vi "File.Sort Path Length, Long to Short.vi"(11 "Path Array":path[](array[path])) -> (3 "Path Array Out":path[](array[path]))   [LabVIEW 2018]
panel:
  # "Longest to Shortest"
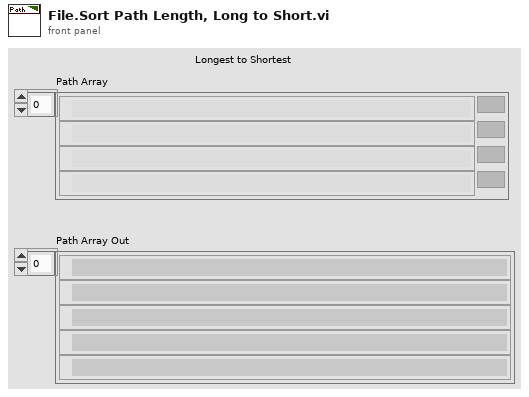
[diagram p1: front panel]
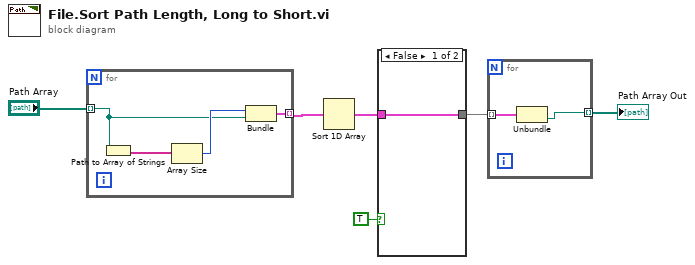
[diagram p0: block diagram]
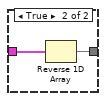
[diagram p2: hidden frame]
diagram:
  n1 = for {
    tunnel: "Path Array" -> [w8] mode=indexing
    tunnel: [w7] -> w5 mode=indexing
    n2 = Path to Array of Strings(0:w8) -> (2:w10:string[])  [unwired: 1 out]
    n3 = Array Size(array=w10) -> (size(s)=w9:i32)
    n4 = Bundle(w9, "Path"=w8) -> (w7:cluster{i32, "Path":path})  [unwired: 1 in]
  }
  n5 = Sort 1D Array(array=w5) -> (sorted array=w4:cluster{i32, "Path":path}[])
  n6 = case shown="False" TRUE {
    tunnel: w4 -> [w11 w13]
    tunnel: [w11 w12] -> w3
    frame False {
    }
    frame True {
      n7 = Reverse 1D Array(array=w13) -> (reversed array=w12:cluster{i32, "Path":path}[])
    }
  }
  n8 = for {
    tunnel: w3 -> [w15] mode=indexing
    tunnel: [w14] -> w2 mode=indexing
    n9 = Unbundle(w15) -> ("Path"=w14:path)  [unwired: 1 out]
  }
  "Path Array Out" <- w2
